vi "Calc Currente Exposure Time.vi"(8 "error in (no error)":errorcluster, 11 "CCDCamera in":refnum<class "Simulated Camera.lvclass">) -> (0 "error out":errorcluster, 3 "CCDCamera out":refnum<class "Simulated Camera.lvclass">)   [LabVIEW 2018, in "Simulated Camera.lvclass"]
doc: "Calculate the exposure time of the current acquisition\n\nThis calculation is based on the timestamp get after the star of the acquisition"
uses:
  Simulated Camera.lvclass
  Simulated Camera.lvclass/Simulated Camera.ctl
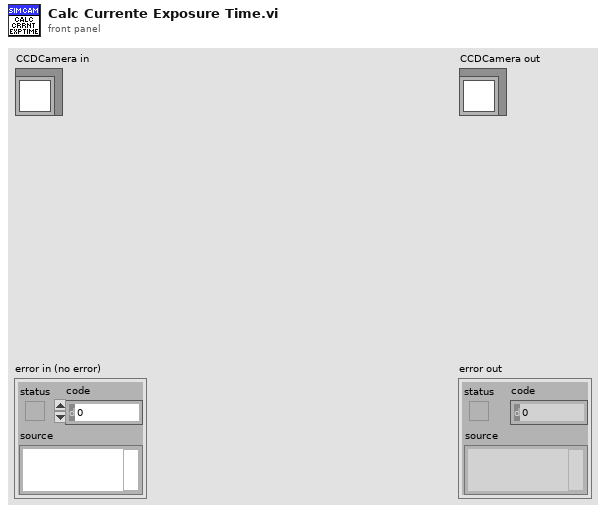
[diagram p1: front panel]
types:
  T1 = cluster{"CYCLES_DONE":u16, "LAST_IMAGE_NAME":string, "DISK_SPACE":u16, "FRAMES_DONE":u16, "CCD_STATUS":string, "CURRENT_TEMPERATURE":i16, "TEMPERATURE_STATUS":string, "FRAME_EXPOSURE_TIME":sgl, "ERROR":bool, "SERIAL_NUMBER":u16, "ACQUIRING":bool, "IMAGE_INDEX":u32, "SEQS_DONE":u16}
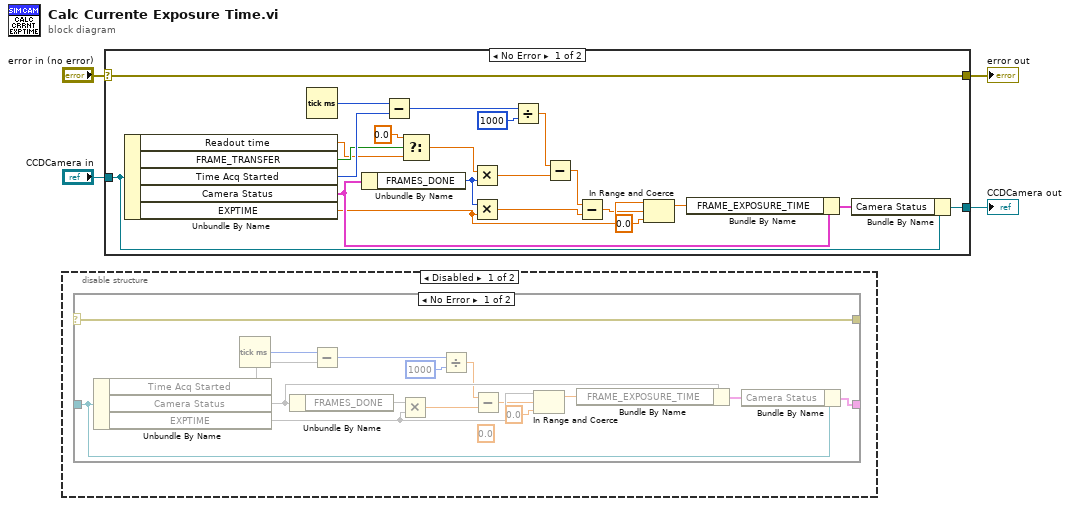
[diagram p0: block diagram]
diagram:
  n1 = disable-structure shown="Disabled" {
    frame Disabled {
      n2 = case shown="No Error" {
        selector: _ -> [w5 w22]
        tunnel: [w5 w22] -> _
        tunnel: [w20 w21] -> _
        tunnel: _ -> [w9 w21]
        frame No Error {
          (unwired) sgl 0.0
          n3 = Unbundle By Name(w9) -> ("Time Acq Started"=w18, "Camera Status"=w15, "EXPTIME"=w13)
          n4 = Tick Count (ms)() -> (millisecond timer value=w19:u32)
          n5 = Unbundle By Name(w15) -> ("FRAMES_DONE"=w6)
          n6 = Subtract(x=w19, y=w18) -> (x-y=w17:u32)
          n7 = Multiply(x=w6, y=w13) -> (x*y=w11:dbl)
          n8 = Divide(x=w17, y=1000) -> (x/y=w7:dbl)
          n9 = Subtract(x=w7, y=w11) -> (x-y=w10:dbl)
          n10 = In Range and Coerce(upper limit=w13, x=w10, lower limit=sgl 0.0) -> (coerced(x)=w8:dbl)  [unwired: 1 out]
          n11 = Bundle By Name(cluster=w15, "FRAME_EXPOSURE_TIME"=w8) -> (w14:cluster{})
          n12 = Bundle By Name(cluster=w9, "Camera Status"=w14) -> (w20:cluster{})
        }
        frame Error {
        }
      }
    }
    frame Enabled {
    }
  }
  n13 = case shown="No Error" "error in (no error)" {
    selector: "error in (no error)" -> [w24 w46]
    tunnel: [w24 w46] -> w2
    tunnel: [w44 w45] -> w1
    tunnel: "CCDCamera in" -> [w31 w45]
    frame No Error {
      n14 = Unbundle By Name(w31) -> ("Readout time"=w23:dbl, "FRAME_TRANSFER"=w32:bool, "Time Acq Started"=w42:u32, "Camera Status"=w39:T1, "EXPTIME"=w37:dbl)
      n15 = Tick Count (ms)() -> (millisecond timer value=w43:u32)
      n16 = Unbundle By Name(w39) -> ("FRAMES_DONE"=w25:u16)
      n17 = Subtract(x=w43, y=w42) -> (x-y=w41:u32)
      n18 = Select(t=sgl 0.0, s=w32, f=w23) -> (s? t:f=w27:dbl)
      n19 = Multiply(x=w27, y=w25) -> (x*y=w26:dbl)
      n20 = Multiply(x=w25, y=w37) -> (x*y=w35:dbl)
      n21 = Divide(x=w41, y=1000) -> (x/y=w29:dbl)
      n22 = Subtract(x=w29, y=w26) -> (x-y=w28:dbl)
      n23 = Subtract(x=w28, y=w35) -> (x-y=w34:dbl)
      n24 = In Range and Coerce(upper limit=w37, x=w34, lower limit=sgl 0.0) -> (coerced(x)=w30:dbl)  [unwired: 1 out]
      n25 = Bundle By Name(cluster=w39, "FRAME_EXPOSURE_TIME"=w30) -> (w38:T1)
      n26 = Bundle By Name(cluster=w31, "Camera Status"=w38) -> (w44:refnum<class "Simulated Camera.lvclass">)
    }
    frame Error {
    }
  }
  "error out" <- w2
  "CCDCamera out" <- w1
